vi "main.vi"() -> ()   [LabVIEW 2018]
doc: "SubVI"
panel:
  in  "Array Out":bool[][](array[boolean])
  in  "Stop":bool
  in  "Open Settings":bool
  # "1. Make sure SubVI is not opened in LabVIEW and that the Index Display of the array is set at (0, 0)\n2. Run main.vi\n3. Open Settings (SubVI front panel is called)\n4. Adjust boolean array\n5. Close SubVI"
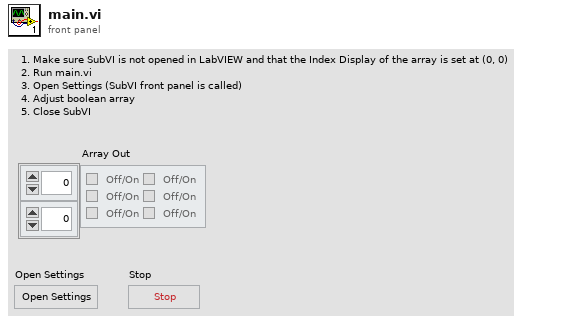
[diagram p1: front panel]
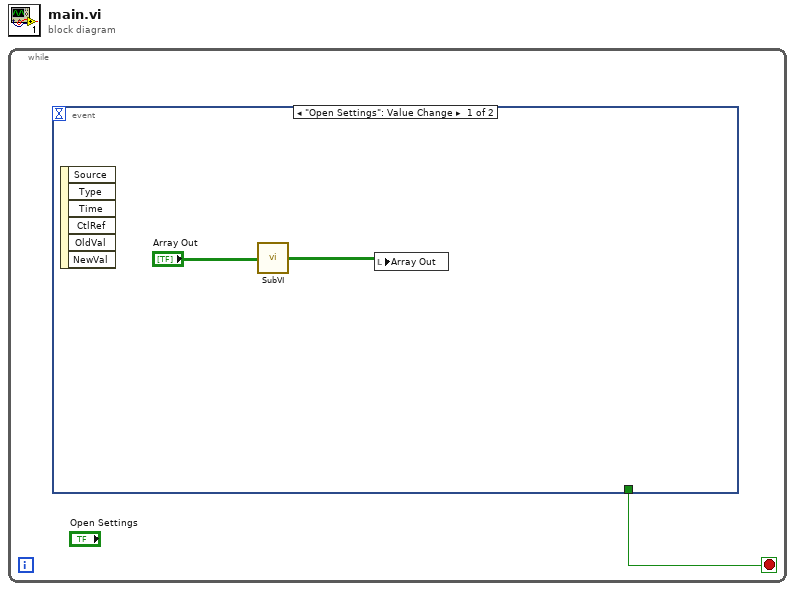
[diagram p0: block diagram]
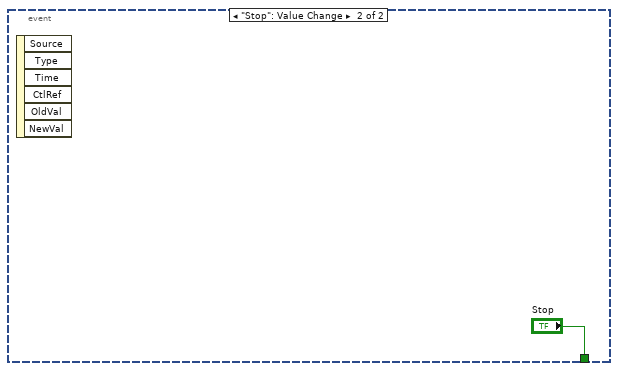
[diagram p2: hidden frame]
diagram:
  n1 = while {
    stop <- w1 stop-if-true
    n2 = event shown="[0] \"Open Settings\": Value Change" {
      selector: _ -> [_ _]
      dyn-events: _ -> [_ _]
      timeout: _ -> [_ _]
      tunnel: [_ "Stop"] -> w1
      event "Open Settings": Value Change {
        n3 = event-data() -> ()  [unwired: 1 in, 6 out]
        n4 = call "SubVI.vi"("Array Control In"="Array Out") -> ("Array Indicator Out"=w2:bool[][])  [unwired: 3 in, 1 out]
        n5 = local write "Array Out"(w2) -> ()
      }
      event "Stop": Value Change {
        n6 = event-data() -> ()  [unwired: 1 in, 6 out]
      }
    }
  }
